vi "Get COM name.vi"(8 "error in (no error)":errorcluster, 11 "VISA resource in":refnum<visa-resource-name>) -> (0 "error IO":errorcluster, 2 "COM name":string, 3 "VISA resource out":refnum<visa-resource-name>)   [LabVIEW 2020, in "Global FIA milliGAT.lvlib"]
uses:
  <instrlib>/RxnRover/Global FIA milliGAT 3.14/Global FIA milliGAT.lvlib
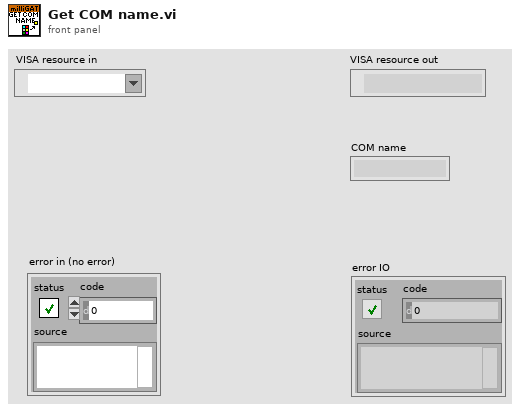
[diagram p1: front panel]
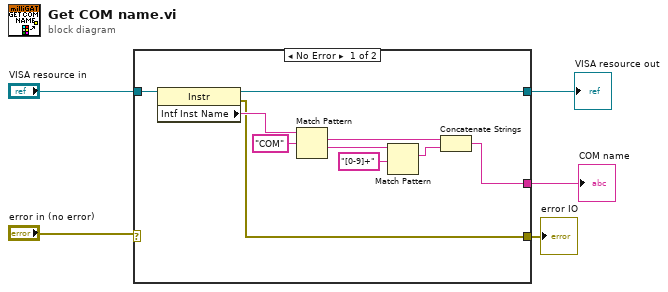
[diagram p0: block diagram]
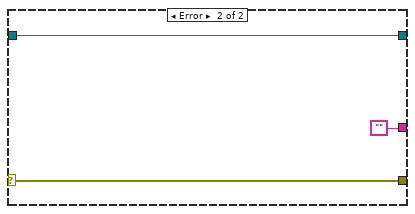
[diagram p2: hidden frame]
diagram:
  n1 = case shown="No Error" "error in (no error)" {
    selector: "error in (no error)" -> [_ w16]
    tunnel: "VISA resource in" -> [w15 w18]
    tunnel: [w9 ""] -> w4
    tunnel: [w8 w18] -> w3
    tunnel: [w6 w16] -> w1
    frame No Error {
      n2 = property class="Instr"(reference=w15) -> (reference out=w8:refnum<visa-resource-name>, error out=w6:errorcluster, "Intf Inst Name"=w14:string)  [unwired: 1 in]
      n3 = Match Pattern(string=w14, regular expression="COM") -> (match substring=w10:string, after substring=w12:string)  [unwired: 1 in, 2 out]
      n4 = Match Pattern(string=w12, regular expression="[0-9]+") -> (match substring=w7:string)  [unwired: 1 in, 3 out]
      n5 = Concatenate Strings(w10, w7) -> (w9:string)
    }
    frame Error {
    }
  }
  "COM name" <- w4
  "VISA resource out" <- w3
  "error IO" <- w1
